vi "Real Dot Product.vi"(2 "Y Vector":dbl[](array[numeric]) format="%.2f", 3 "X Vector":dbl[](array[numeric]) format="%.2f") -> (0 "error":i32, 1 "X * Y":dbl format="%.2f")   [LabVIEW 2024, in "NI_AALBase.lvlib"]
doc: "<p>Computes the dot product of <strong>X Vector</strong> and <strong>Y Vector</strong>. The data types you wire to the <strong>X Vector</strong> and <strong>Y Vector</strong> inputs determine the polymorphic instance to use.</p>"
uses:
  NI_AALBase.lvlib
  <resource>/lvanlys.dll
panel:
  # "Dot Product"
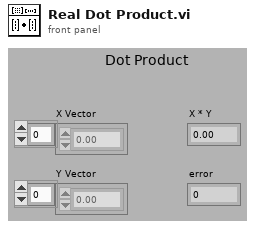
[diagram p1: front panel]
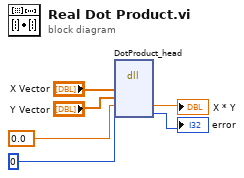
[diagram p0: block diagram]
diagram:
  n1 = dll-call lib="C:/Program Files (x86)/National Instruments/LabVIEW 2024/resource/lvanlys.*" fn="DotProduct_head"("X Vector"="X Vector", "Y Vector"="Y Vector", 0.0, 0) -> (→"X * Y":dbl, →"error":i32)  [unwired: 6 in, 2 out]
